vi "GEM_BANK_Get_Entries.vi"(8 "error in (no error)":errorcluster, 11 "LVBANK in":refnum<class "GEM_BANK.lvclass">) -> (0 "error out":errorcluster, 2 "Count of LVDATA":i32, 3 "LVBANK out":refnum<class "GEM_BANK.lvclass">)   [LabVIEW 2018, in "feGEM DataPacker.lvlib" / "GEM_BANK.lvclass"]
uses:
  GEM_BANK.lvclass
  GEM_BANK.lvclass/GEM_BANK.ctl
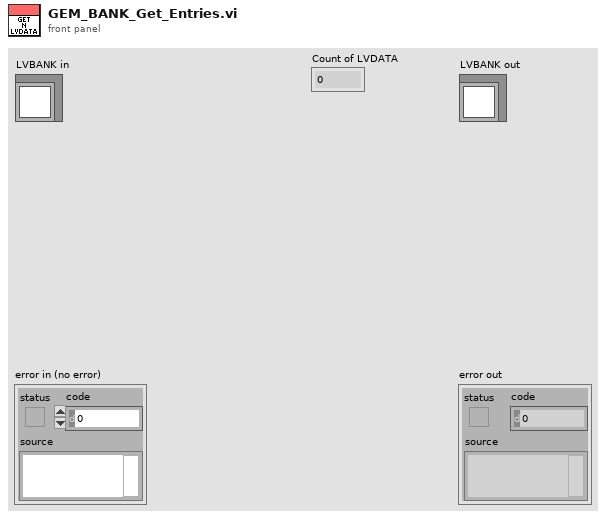
[diagram p1: front panel]
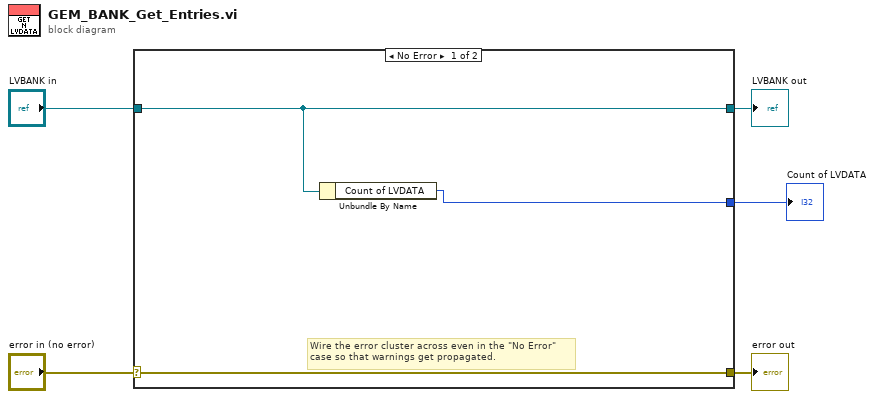
[diagram p0: block diagram]
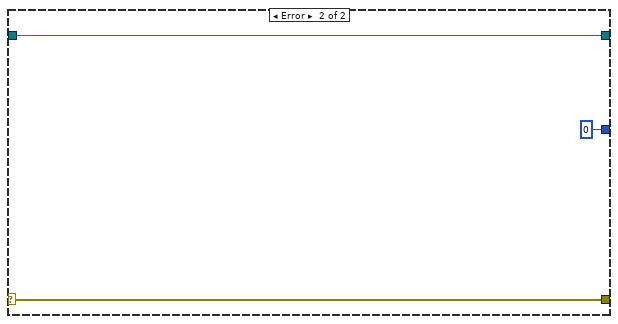
[diagram p2: hidden frame]
diagram:
  n1 = case shown="No Error" "error in (no error)" {
    selector: "error in (no error)" -> [w8 w11]
    tunnel: [w8 w11] -> w4
    tunnel: [w7 w10] -> w2
    tunnel: "LVBANK in" -> [w7 w10]
    tunnel: [w6 0 ("Count of LVDATA")] -> w1
    frame No Error {
      # "Wire the error cluster across even in the \"No Error\"\ncase so that warnings get propagated."
      n2 = Unbundle By Name(w7) -> ("Count of LVDATA"=w6:i32)
    }
    frame Error {
    }
  }
  "error out" <- w4
  "LVBANK out" <- w2
  "Count of LVDATA" <- w1
